vi "Actor Launched.vi"(5 "Actor Type":string, 7 "Actor Core VI":string, 8 "error in (no error)":errorcluster, 9 "Actor's Caller Q":refnum<class "Message Enqueuer.lvclass">, 10 "Actor's Self Q":refnum<class "Message Enqueuer.lvclass">, 11 "Monitor Data in":refnum<class "Monitor Data.lvclass">) -> (0 "error out":errorcluster, 3 "Monitor Data out":refnum<class "Monitor Data.lvclass">)   [LabVIEW 2023, in "Monitored Actor.lvlib" / "Monitor Data.lvclass"]
doc: "Add the new actor to the data store\n\nCopyright: MGI 2016\nAuthor: Derek Trepanier"
uses:
  Monitor Data.lvclass
  builds/Engine/Actor Framework.lvlibp/1abvi3w/vi.lib/ActorFramework/Message Enqueuer/Message Enqueuer.lvclass
  Monitor Data.lvclass/Monitor Data.ctl
  Actor Data.ctl
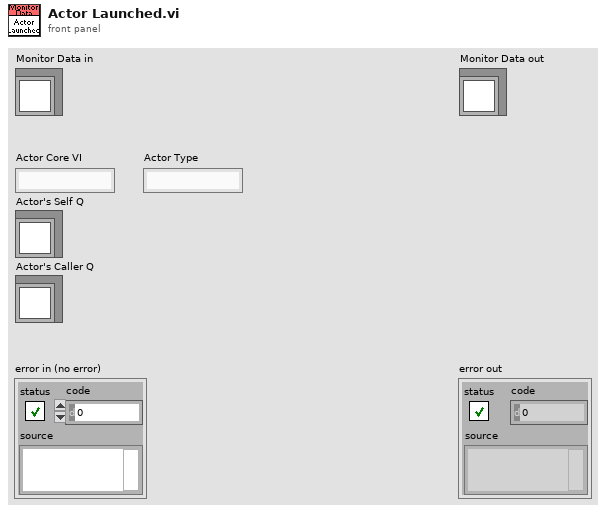
[diagram p1: front panel]
types:
  T1 = typedef "Monitored Actor.lvlib/Monitor Data.lvclass/Actor Data.ctl" = cluster{"Actor Type":string, "Actor Core VI":string, "Self":refnum<class "Message Enqueuer.lvclass">, "Caller":refnum<class "Message Enqueuer.lvclass">, "Actor Label":string, "Last Ping":dbl}
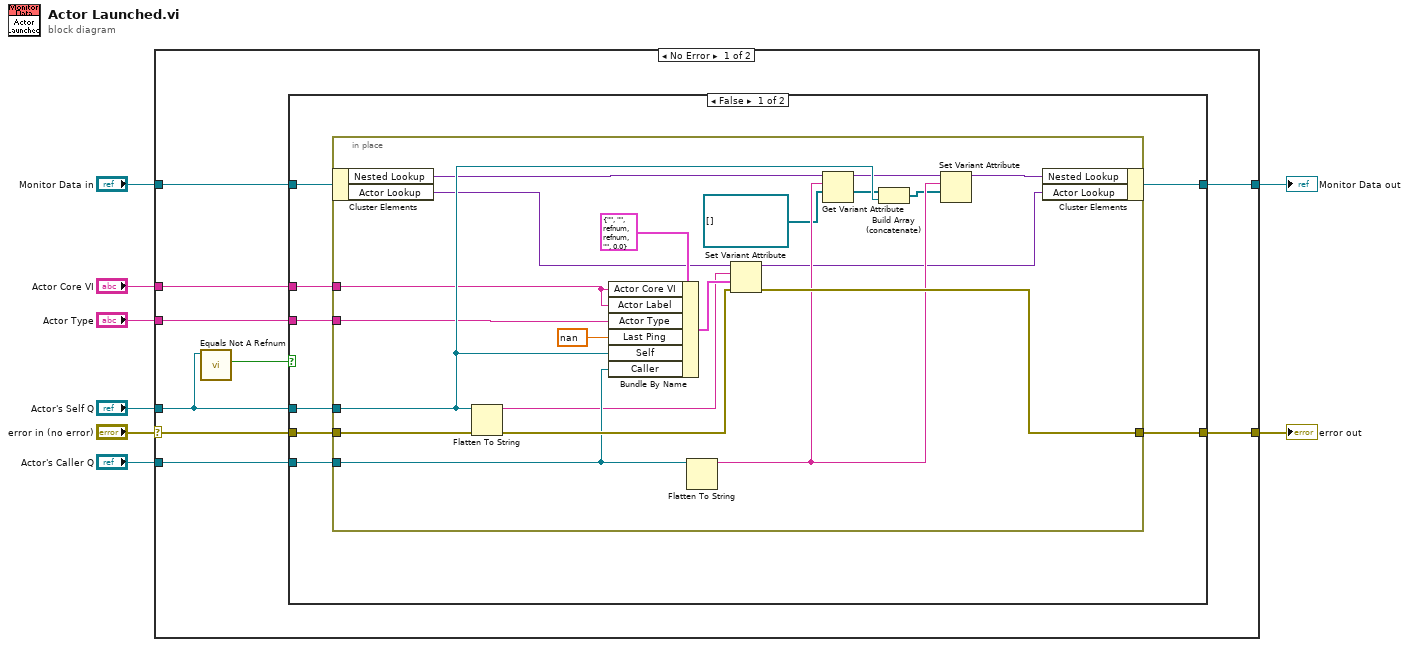
[diagram p0: block diagram]
diagram:
  n1 = case shown="No Error" "error in (no error)" {
    selector: "error in (no error)" -> [w12 w49]
    tunnel: [w13 w49] -> w6
    tunnel: [w14 w48] -> w7
    tunnel: "Monitor Data in" -> [w15 w48]
    tunnel: "Actor's Self Q" -> [w10 _]
    tunnel: "Actor Core VI" -> [w17 _]
    tunnel: "Actor's Caller Q" -> [w16 _]
    tunnel: "Actor Type" -> [w11 _]
    frame No Error {
      n2 = call "Equals Not A Refnum.vi"("Message Enqueuer"=w10) -> ("Not a refnum?"=w9:bool)  [unwired: 10 in]
      n3 = case shown="False" w9 {
        tunnel: w10 -> [w25 _]
        tunnel: w17 -> [w24 _]
        tunnel: w16 -> [w23 _]
        tunnel: w15 -> [w22 w47]
        tunnel: [w21 w47] -> w14
        tunnel: [w20 w46] -> w13
        tunnel: w12 -> [w19 w46]
        tunnel: w11 -> [w18 _]
        frame False {
          n4 = in-place {
            in-place-border: w25 -> [w40]
            in-place-border: [w43] -> w20
            in-place-border: w24 -> [w28]
            in-place-border: w23 -> [w42]
            in-place-border: w19 -> [w30]
            in-place-border: w18 -> [w27]
            n5 = in-place-cluster #1(w22) -> ("Nested Lookup"=w32:variant, "Actor Lookup"=w34:variant)
            n6 = Flatten To String(anything=w40, error in (no error)=w30) -> (data string=w26:string, error out=w45:errorcluster)  [unwired: 2 in, 1 out]
            n7 = Bundle By Name(cluster=T1 {"Actor Type"="", "Actor Core VI"="", "Self"=refnum, "Caller"=refnum, "Actor Label"="", "Last Ping"=0.0} ("Actor Data"), "Actor Core VI"=w28, "Actor Label"=w28, "Actor Type"=w27, "Last Ping"=nan, "Self"=w40, "Caller"=w42) -> (w44:T1)
            n8 = Flatten To String(anything=w42) -> (data string=w39:string)  [unwired: 3 in, 2 out]
            n9 = Set Variant Attribute(Variant=w34, name=w26, value=w44, error in=w45) -> (Variant out=w33:variant, error out=w43:errorcluster)  [unwired: 1 out]
            n10 = Get Variant Attribute(Variant=w32, name=w39, default value (empty Variant)=refnum<class "Message Enqueuer.lvclass">[] []) -> (duplicate Variant=w36:variant, value=w37:refnum<class "Message Enqueuer.lvclass">[])  [unwired: 1 in, 2 out]
            n11 = Build Array (concatenate)(w37, w40) -> (w35:refnum<class "Message Enqueuer.lvclass">[])
            n12 = Set Variant Attribute(Variant=w36, name=w39, value=w35) -> (Variant out=w31:variant)  [unwired: 1 in, 2 out]
            n13 = in-place-cluster #1("Nested Lookup"=w31, "Actor Lookup"=w33) -> (w21:refnum<class "Monitor Data.lvclass">)
          }
        }
        frame True {
        }
      }
    }
    frame Error {
    }
  }
  "error out" <- w6
  "Monitor Data out" <- w7
